vi "set_Period_subvi.vi"(7 "Period":dbl, 8 "error in (no error)":errorcluster, 9 "Aardvark Handle":i32 min=0, 10 "Num Bytes to Fetch (64) in":u16=64 min=1, 11 "Address (0x50) in":u16=80 max=1023 format="%.0x") -> (0 "error out":errorcluster)   [LabVIEW 2014]
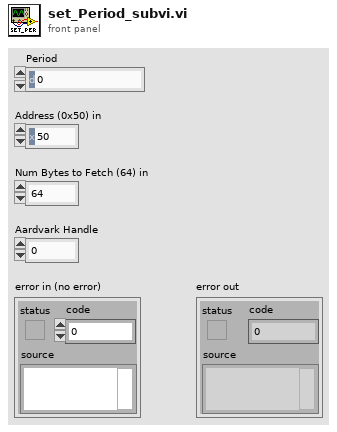
[diagram p1: front panel]
types:
  T1 = cluster{"unsigned byte array[0]":u8, "unsigned byte array[1]":u8, "unsigned byte array[2]":u8, "unsigned byte array[3]":u8, "unsigned byte array[4]":u8, "unsigned byte array[5]":u8, "unsigned byte array[6]":u8, "unsigned byte array[7]":u8, "unsigned byte array[8]":u8}
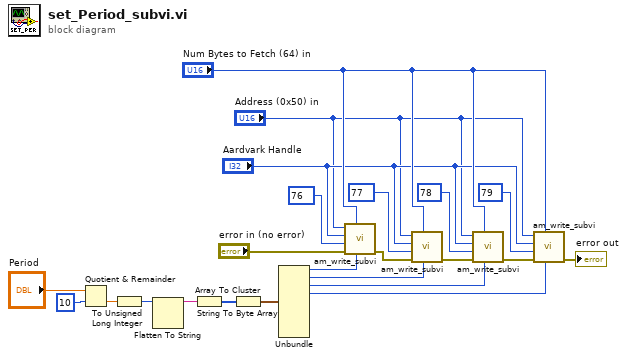
[diagram p0: block diagram]
diagram:
  n1 = Quotient & Remainder(x="Period", y=10) -> (floor(x/y)=w4:dbl)  [unwired: 1 out]
  n2 = To Unsigned Long Integer(number=w4) -> (unsigned 32bit integer=w5:u32)
  n3 = Flatten To String(anything=w5) -> (data string=w3:string)  [unwired: 3 in, 2 out]
  n4 = String To Byte Array(string=w3) -> (unsigned byte array=w6:u8[])
  n5 = Array To Cluster(array=w6) -> (cluster=w7:T1)
  n6 = Unbundle(w7) -> ("unsigned byte array[0]"=w20:u8, "unsigned byte array[1]"=w21:u8, "unsigned byte array[2]"=w22:u8, "unsigned byte array[3]"=w23:u8)  [unwired: 5 out]
  n7 = call "am_write_subvi.vi"("Data to Write"=w20, "Num Bytes to Fetch (64)"="Num Bytes to Fetch (64) in", "error in (no error)"="error in (no error)", "Memory ADD"=u16 76, "Aardvark Handle in"="Aardvark Handle", "Address (0x50) in"="Address (0x50) in") -> ("error out"=w9:errorcluster)  [unwired: 4 in, 1 out]
  n8 = call "am_write_subvi.vi"("Data to Write"=w21, "Num Bytes to Fetch (64)"="Num Bytes to Fetch (64) in", "error in (no error)"=w9, "Memory ADD"=u16 77, "Aardvark Handle in"="Aardvark Handle", "Address (0x50) in"="Address (0x50) in") -> ("error out"=w10:errorcluster)  [unwired: 4 in, 1 out]
  n9 = call "am_write_subvi.vi"("Data to Write"=w22, "Num Bytes to Fetch (64)"="Num Bytes to Fetch (64) in", "error in (no error)"=w10, "Memory ADD"=u16 78, "Aardvark Handle in"="Aardvark Handle", "Address (0x50) in"="Address (0x50) in") -> ("error out"=w11:errorcluster)  [unwired: 4 in, 1 out]
  n10 = call "am_write_subvi.vi"("Data to Write"=w23, "Num Bytes to Fetch (64)"="Num Bytes to Fetch (64) in", "error in (no error)"=w11, "Memory ADD"=u16 79, "Aardvark Handle in"="Aardvark Handle", "Address (0x50) in"="Address (0x50) in") -> ("error out"=→"error out":errorcluster)  [unwired: 4 in, 1 out]
